vi "Database Delete.vi"() -> ()   [LabVIEW 2023]
doc: "This example demonstrates how to use the DB Tools Delete Data VI to delete specific data from a database, located at LabVIEW\\examples\\database\\LabVIEW.mdb.\n\nThis example first creates a table, named DeleteData, in the database and inserts some randomly generated numbers to the table. This example then uses the DB Tools Delete Data VI to delete all numbers that equal the numeric value 1. The <B>Before</B> and <B>After</B> arrays display the original data and the remaining data, respectively."
uses:
  <vilib>/addons/database/Connection.llb/DB Tools Open Connec (Path).vi
  <vilib>/addons/database/_DB Variant To Data/Database Variant To Data.xnode
  <vilib>/addons/database/NI_Database_API.lvlib
panel:
  out "After":string[][](array[string])
  out "Before":string[][](array[string])
  # "Overview: Demonstrates how to delete data from a database.\nRequirements: Database Connectivity Toolkit\nInstructions:\nRun the VI to display Before and After data from the database table. All values that equal \"1\" are removed."
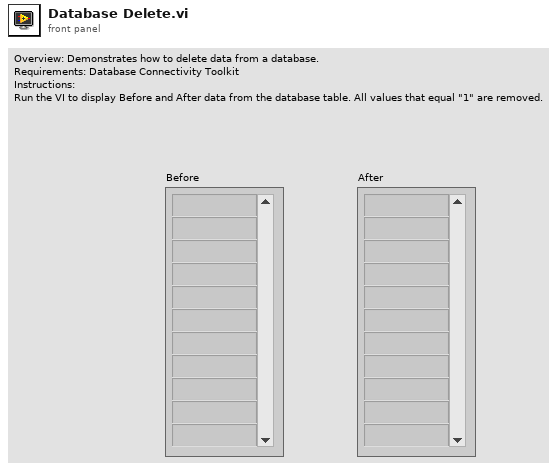
[diagram p1: front panel]
types:
  T1 = typedef "NI_Database_API.lvlib/Conn ObjectReference.ctl" = refnum<k1>
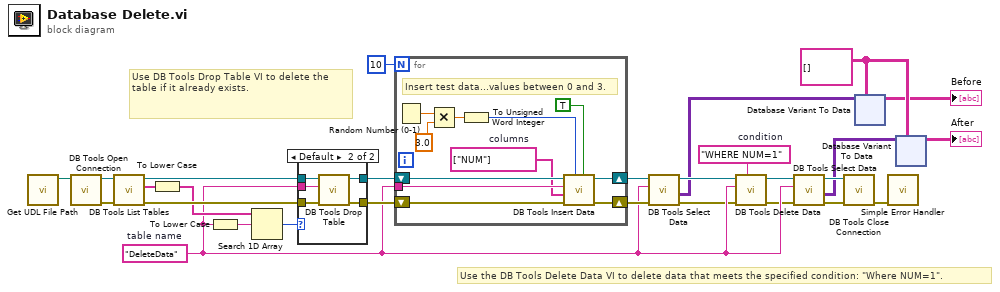
[diagram p0: block diagram]
diagram:
  w4 = string[][] []
  w7 = "WHERE NUM=1"  # condition
  w11 = "DeleteData"  # table name
  # "Use the DB Tools Delete Data VI to delete data that meets the specified condition: \"Where NUM=1\"."
  # "Use DB Tools Drop Table VI to delete the table if it already exists."
  n1 = call "Get UDL File Path.vi"() -> ("UDL file path"=w12:path)  [unwired: 11 in]
  n2 = call-poly <vilib>:"DB Tools Open Connection.vi"("connection information"=w12) -> ("error out"=w15:errorcluster, "connection reference"=w16:T1)  [unwired: 7 in]
  n3 = call <vilib>:"DB Tools List Tables.vi"("error in (no error)"=w15, "connection reference"=w16) -> ("error out"=w21:errorcluster, "tables"=w20:string[], "connection reference out"=w22:T1)  [unwired: 3 in]
  n4 = To Lower Case(string=w20) -> (all lower case string=w18:string[])
  n5 = To Lower Case(string=w11) -> (all lower case string=w19:string)
  n6 = Search 1D Array(1D array=w18, element=w19) -> (index of element=w17:i32)  [unwired: 1 in]
  n7 = case shown="Default" w17 {
    tunnel: w21 -> [w29 w35]
    tunnel: w22 -> [w30 w34]
    tunnel: [w30 w33] -> w14
    tunnel: [w29 w32] -> w13
    tunnel: w11 -> [_ w31]
    frame -1 {
    }
    frame Default {
      n8 = call <vilib>:"DB Tools Drop Table.vi"("error in (no error)"=w35, "table"=w31, "connection reference"=w34) -> ("error out"=w32:errorcluster, "connection reference out"=w33:T1)  [unwired: 5 in]
    }
  }
  n9 = for {
    N: 10 -> [_]
    shift-right: [w45] -> w25
    shift-left: w13 -> [w46]
    tunnel: w11 -> [w38]
    shift-right: [w44] -> w24
    shift-left: w14 -> [w39]
    w36 = string[] ["NUM"]  # columns
    # "Insert test data...values between 0 and 3."
    n10 = Random Number (0-1)() -> (number: 0 to 1=w42:dbl)
    n11 = Multiply(x=w42, y=3.0) -> (x*y=w40:dbl)
    n12 = To Unsigned Word Integer(number=w40) -> (unsigned 16bit integer=w37:u16)
    n13 = call <vilib>:"DB Tools Insert Data.vi"("create table? (F)"=TRUE ("create table? (f)"), "data"=w37, "error in (no error)"=w46, "columns"=w36, "table"=w38, "connection reference"=w39) -> ("error out"=w45:errorcluster, "connection reference out"=w44:T1)  [unwired: 4 in]
  }
  n14 = call <vilib>:"DB Tools Select Data.vi"("error in (no error)"=w25, "table"=w11, "connection reference"=w24) -> ("error out"=w1:errorcluster, "data"=w6:variant[][], "connection reference out"=w8:T1)  [unwired: 3 in]
  n15 = call <vilib>:"DB Tools Delete Data.vi"("condition"=w7, "error in (no error)"=w1, "table"=w11, "connection reference"=w8) -> ("error out"=w9:errorcluster, "connection reference out"=w10:T1)  [unwired: 6 in]
  n16 = call <vilib>:"DB Tools Select Data.vi"("error in (no error)"=w9, "table"=w11, "connection reference"=w10) -> ("error out"=w27:errorcluster, "data"=w5:variant[][], "connection reference out"=w28:T1)  [unwired: 3 in]
  n17 = call <vilib>:"DB Tools Close Connection.vi"("error in (no error)"=w27, "connection reference"=w28) -> ("error out"=w26:errorcluster)  [unwired: 5 in]
  n18 = xnode "Database Variant To Data"("database variant"=w6, "type"=w4) -> ("data"=→"Before":string[][])  [unwired: 1 in, 1 out]
  n19 = call <vilib>:"Simple Error Handler.vi"("error in (no error)"=w26) -> ()  [unwired: 4 in, 5 out]
  n20 = xnode "Database Variant To Data"("database variant"=w5, "type"=w4) -> ("data"=→"After":string[][])  [unwired: 1 in, 1 out]
